vi "Custom_NOT.vi"(11 "Input":bool) -> (3 "Output":bool)   [LabVIEW 2026]
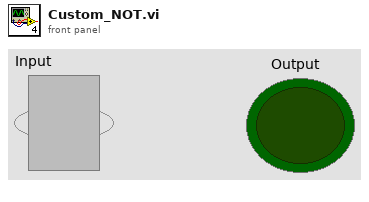
[diagram p1: front panel]
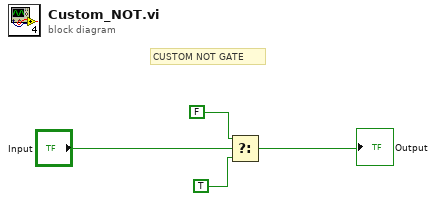
[diagram p0: block diagram]
diagram:
  # "CUSTOM NOT GATE"
  n1 = Select(t=FALSE, s="Input", f=TRUE) -> (s? t:f=→"Output":bool)
